vi "WaitFirstRes.vi"(8 "error in (no error)":errorcluster, 11 "VISA in":refnum<visa-resource-name>) -> (0 "error out":errorcluster, 1 "String":string, 2 "Version":string, 3 "VISA out":refnum<visa-resource-name>, 4 "RespTime":u32, 5 "Local Origin":cluster{"X":dbl, "Y":dbl, "Z":dbl})   [LabVIEW 2022 SP3]
panel:
  out "remaining string":string
  out "after substring":string
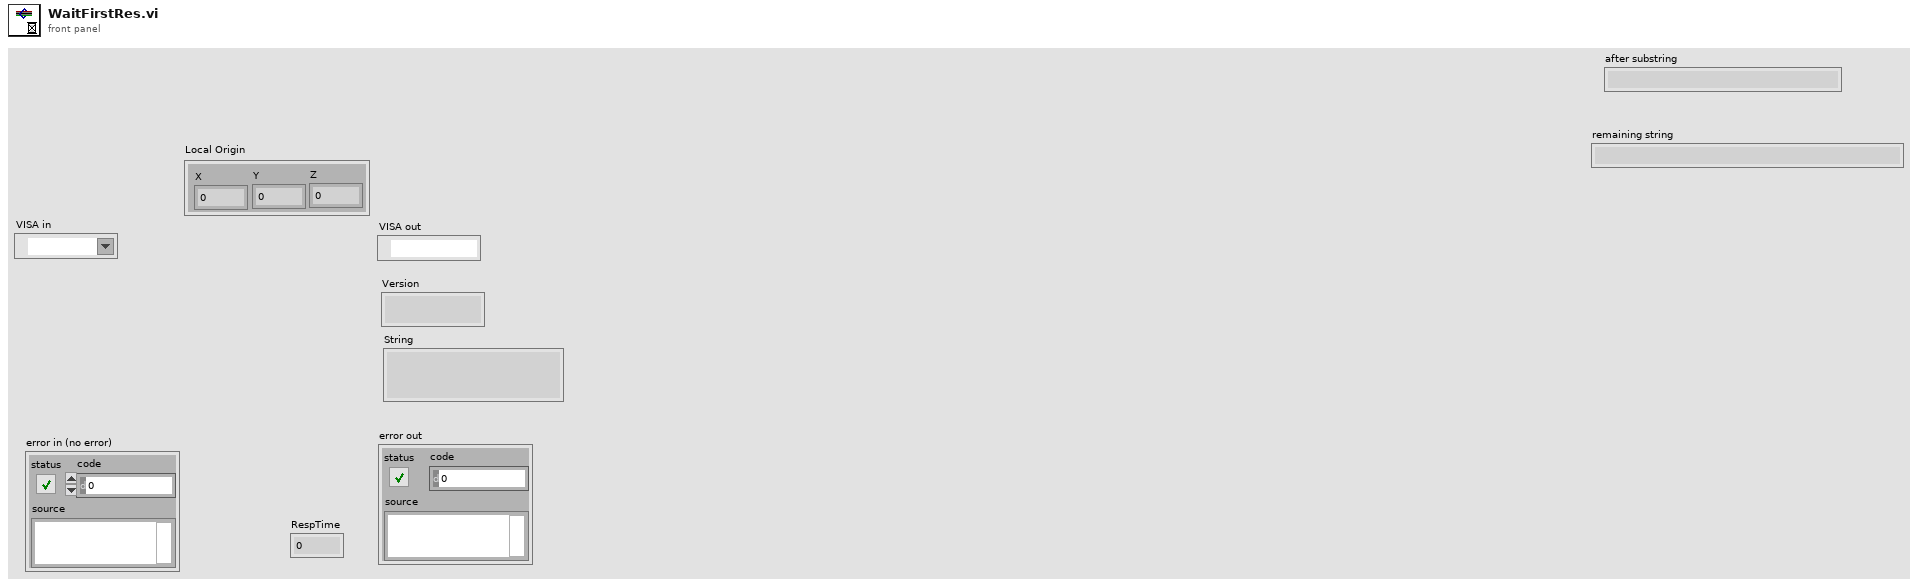
[diagram p1: front panel]
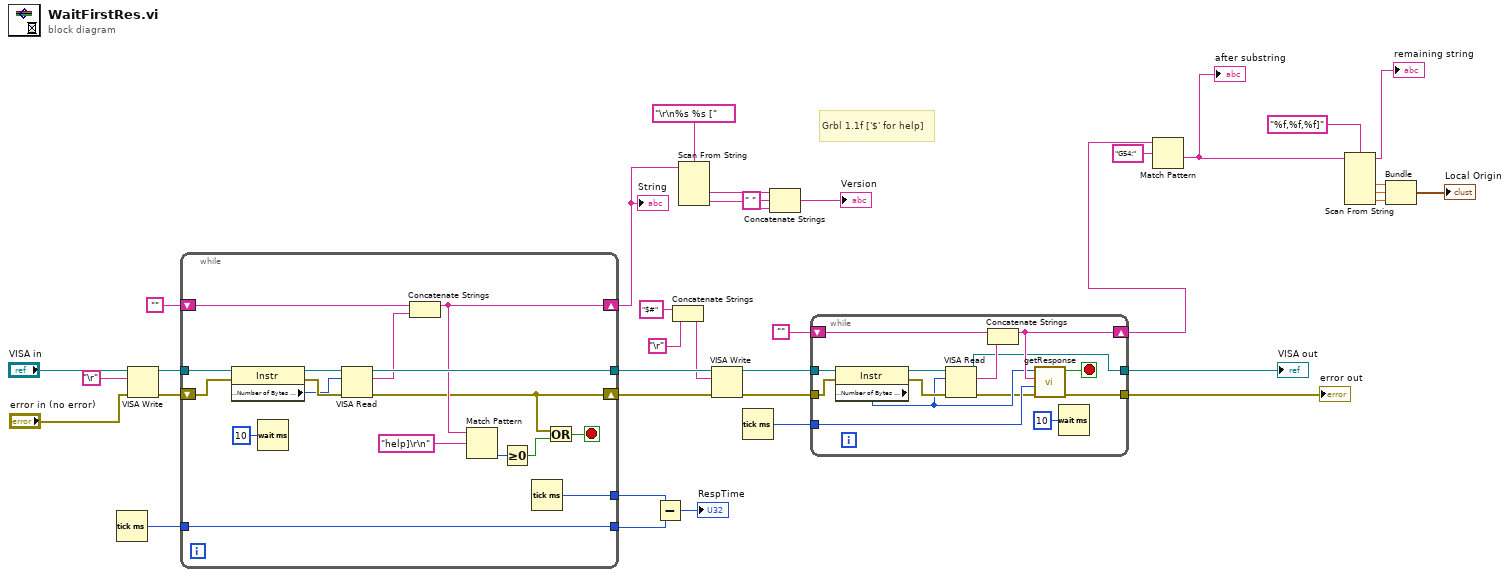
[diagram p0: block diagram]
diagram:
  # "Grbl 1.1f ['$' for help]"
  n1 = Tick Count (ms)() -> (millisecond timer value=w30:u32)
  n2 = VISA Write(VISA resource name="VISA in", write buffer="\r", error in (no error)="error in (no error)") -> (VISA resource name out=w35:refnum<visa-resource-name>, error out=w34:errorcluster)  [unwired: 1 out]
  n3 = while {
    tunnel: w35 -> [w51]
    shift-right: [w41] -> w19
    shift-left: w34 -> [w50]
    tunnel: [w47] -> w20
    shift-right: [w43] -> w25
    shift-left: "" -> [w46]
    tunnel: [w38] -> w29
    tunnel: [w37] -> w28
    tunnel: w30 -> [w37]
    stop <- w39 stop-if-true
    n4 = property class="Instr"(reference=w51, error in=w50) -> (reference out=w52:refnum<visa-resource-name>, error out=w53:errorcluster, "Serial Settings:Number of Bytes at Serial Port"=w48:u32)
    n5 = Wait (ms)(milliseconds to wait=u32 10) -> ()  [unwired: 1 out]
    n6 = VISA Read(VISA resource name=w52, byte count=w48, error in (no error)=w53) -> (VISA resource name out=w47:refnum<visa-resource-name>, read buffer=w45:string, error out=w41:errorcluster)  [unwired: 1 out]
    n7 = Concatenate Strings(w46, w45) -> (w43:string)
    n8 = Match Pattern(string=w43, regular expression="help]\r\n" ("response")) -> (offset past match=w42:i32)  [unwired: 1 in, 3 out]
    n9 = Greater Or Equal To 0?(x=w42) -> (x >= 0?=w40:bool)
    n10 = Tick Count (ms)() -> (millisecond timer value=w38:u32)
    n11 = Or(x=w41, y=w40) -> (x .or. y?=w39:bool)
  }
  "String" <- w25
  n12 = Subtract(x=w29, y=w28) -> (x-y=→"RespTime":u32)
  n13 = Concatenate Strings("$#" ("string"), "\r") -> (w16:string)
  n14 = Scan From String(format string="\r\n%s %s [", input string=w25) -> (output 1=w24:string, output 2=w22:string)  [unwired: 4 in, 3 out]
  n15 = VISA Write(VISA resource name=w20, write buffer=w16, error in (no error)=w19) -> (VISA resource name out=w15:refnum<visa-resource-name>, error out=w14:errorcluster)  [unwired: 1 out]
  n16 = Tick Count (ms)() -> (millisecond timer value=w12:u32)
  n17 = Concatenate Strings(w24, " " ("string"), w22) -> (→"Version":string)
  n18 = while {
    tunnel: w15 -> [w67]
    tunnel: w14 -> [w55]
    shift-right: [w62] -> w3
    shift-left: "" -> [w64]
    tunnel: [w54] -> w11
    tunnel: [w57] -> w10
    tunnel: w12 -> [w61]
    stop <- w59 stop-if-true
    n19 = property class="Instr"(reference=w67, error in=w55) -> (reference out=w65:refnum<visa-resource-name>, error out=w66:errorcluster, "Serial Settings:Number of Bytes at Serial Port"=w60:u32)
    n20 = VISA Read(VISA resource name=w65, byte count=w60, error in (no error)=w66) -> (VISA resource name out=w54:refnum<visa-resource-name>, read buffer=w63:string, error out=w58:errorcluster)  [unwired: 1 out]
    n21 = Concatenate Strings(w64, w63) -> (w62:string)
    n22 = call "getResponse.vi"("error in (no error)"=w58, "ST"=w61, "string"=w62, "Bytes at Serial Port"=w60) -> ("error out"=w57:errorcluster, "done"=w59:bool)  [unwired: 5 in, 1 out]
    n23 = Wait (ms)(milliseconds to wait=u32 10) -> ()  [unwired: 1 out]
  }
  "VISA out" <- w11
  "error out" <- w10
  n24 = Match Pattern(string=w3, regular expression="G54:") -> (after substring=w8:string)  [unwired: 1 in, 3 out]
  "after substring" <- w8
  n25 = Scan From String(format string="%f,%f,%f]", input string=w8) -> (remaining string=→"remaining string":string, output 1=w6:dbl, output 2=w4:dbl, output 3=w5:dbl)  [unwired: 5 in, 2 out]
  n26 = Bundle(w6, w4, w5) -> (→"Local Origin":cluster{dbl, dbl, dbl})  [unwired: 1 in]
